vi "change_phase_array.vi"(8 "frekans":dbl, 9 "index r":dbl, 10 "Change Phase":dbl, 11 "Base Array":dbl[][](array[numeric])) -> (3 "output array":dbl[][](array[numeric]))   [LabVIEW 2014]
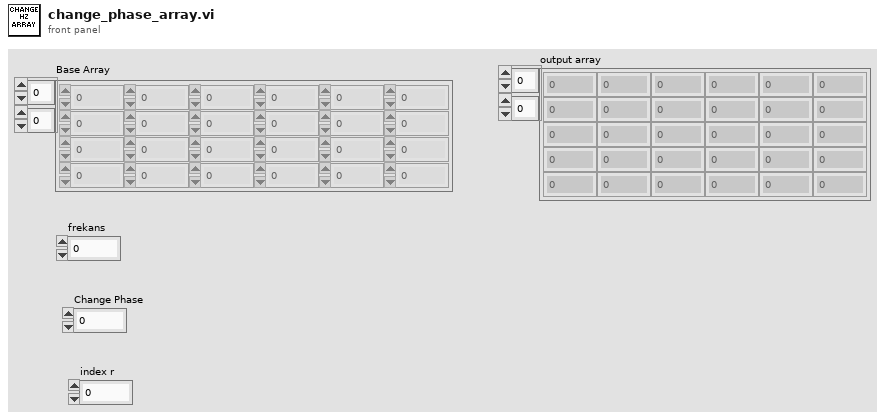
[diagram p1: front panel]
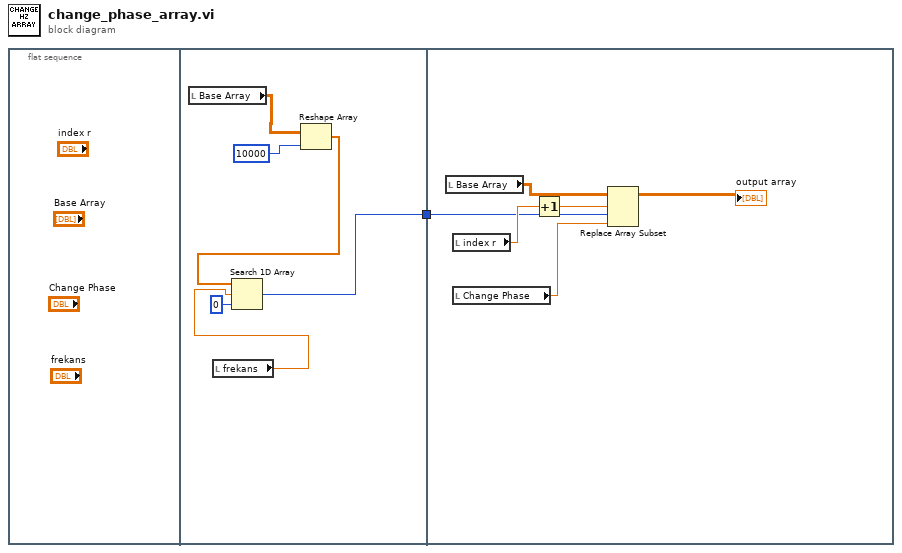
[diagram p0: block diagram]
diagram:
  n1 = flat-sequence {
    tunnel: [w4] -> w1
    tunnel: w1 -> [w11]
    frame #0 {
    }
    frame #1 {
      n2 = local read "Base Array"() -> (w7:dbl[][])
      n3 = local read "frekans"() -> (w3:dbl)
      n4 = Reshape Array(w7, 10000 ("dimension size")) -> (w6:dbl[])
      n5 = Search 1D Array(1D array=w6, element=w3, start index (0)=0) -> (index of element=w4:i32)
    }
    frame #2 {
      n6 = local read "Base Array"() -> (w13:dbl[][])
      n7 = local read "index r"() -> (w12:dbl)
      n8 = local read "Change Phase"() -> (w10:dbl)
      n9 = Increment(x=w12) -> (x+1=w8:dbl)
      n10 = Replace Array Subset(array=w13, new element=w10, index (row)=w8, index (col)=w11) -> (→"output array":dbl[][])
    }
  }
